vi "reset manipulator.vi"(8 "error in":errorcluster, 9 "approach? (T = on)":bool, 10 "motion":T1=enum."slow_dualPatch", 11 "manip in":T2={"Actuator COM"="COM14", "Actuator type"=enum."Scientifica"}) -> (0 "error out":errorcluster, 3 "manip out":T2={"Actuator COM"="COM14", "Actuator type"=enum."Scientifica"})   [LabVIEW 2015]
uses:
  pipette cleaning/pressure box/cleaning_soft/controls/actuator_type.ctl
  pipette cleaning/pressure box/cleaning_soft/controls/actuator_cluster.ctl
  controls/scope_motion.ctl
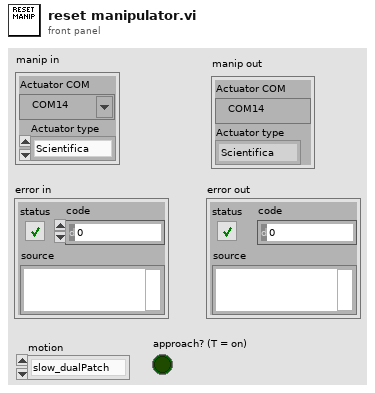
[diagram p1: front panel]
types:
  T1 = typedef "scope_motion.ctl" = enum16{"superSlow", "fast", "slow", "find slice speed", "slow_dualPatch"}
  T2 = typedef "actuator_cluster.ctl" = cluster{"Actuator COM":refnum<visa-resource-name>, "Actuator type":T3}
  T3 = typedef "actuator_type.ctl" = enum16{"Scientifica", "Sutter", "Demo", "Off"}
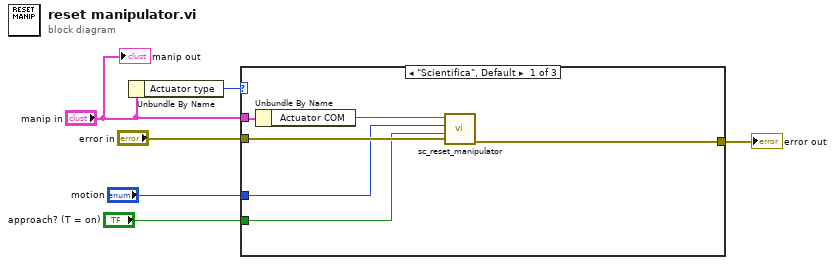
[diagram p0: block diagram]
diagram:
  n1 = Unbundle By Name("manip in") -> ("Actuator type"=w6:T3)
  n2 = case shown="\"Scientifica\", Default" w6 {
    tunnel: "manip in" -> [w12 _ _]
    tunnel: "error in" -> [w10 w13 w14]
    tunnel: [w9 w13 w14] -> w3
    tunnel: "approach? (T = on)" -> [w8 _ _]
    tunnel: "motion" -> [w7 _ _]
    frame "Scientifica", Default {
      n3 = Unbundle By Name(w12) -> ("Actuator COM"=w11:refnum<visa-resource-name>)
      n4 = call "sc_reset_manipulator.vi"("error in (no error)"=w10, "approach? (T = on)"=w8, "motion"=w7, "visa in"=w11) -> ("error out"=w9:errorcluster)  [unwired: 6 in, 1 out]
    }
    frame "Sutter" {
    }
    frame "Demo" {
    }
  }
  "error out" <- w3
  "manip out" <- "manip in"
